vi "Search Hovered Shape.vi"(8 "error in (no error)":errorcluster, 10 "Coords":T1, 11 "Image Editor Handler in":refnum<class "Image Editor Handler.lvclass">) -> (0 "error out":errorcluster, 2 "Node ID":i32, 3 "Image Editor Handler out":refnum<class "Image Editor Handler.lvclass">)   [LabVIEW 2017, in "LV Image Editor Framework.lvlib" / "Image Editor Handler.lvclass"]
uses:
  <vilib>/LIEF/Image Editor Handler/Image Editor Handler.lvclass
  <vilib>/Utility/miscctls.llb/LVPoint32TypeDef.ctl
  <vilib>/LIEF/Image Editor Handler/Image Editor Handler.lvclass/Image Editor Handler.ctl
  <vilib>/LIEF/Forms/Shape/Shape.lvclass
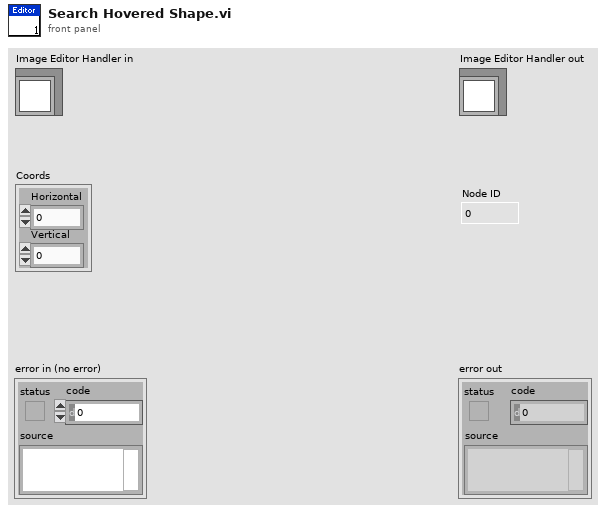
[diagram p1: front panel]
types:
  T1 = typedef "LVPoint32TypeDef.ctl" = cluster{"Horizontal":i32, "Vertical":i32}
  T2 = typedef "LVPositionTypeDef.ctl" = cluster{"Left":i32, "Top":i32}
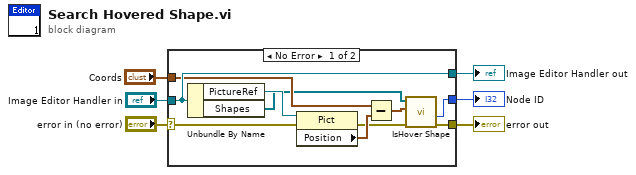
[diagram p0: block diagram]
diagram:
  n1 = case shown="No Error" "error in (no error)" {
    selector: "error in (no error)" -> [w7 w18]
    tunnel: [w10 w18] -> w5
    tunnel: [w16 w17] -> w3
    tunnel: "Image Editor Handler in" -> [w16 w17]
    tunnel: "Coords" -> [w14 _]
    tunnel: [w9 _] -> w1
    frame No Error {
      n2 = Unbundle By Name(w16) -> ("PictureRef"=w15:refnum<vi>, "Shapes"=w12:refnum<data-value>[])
      n3 = property class="Pict"(reference=w15, error in=w7) -> (error out=w8:errorcluster, "Position"=w13:T2)  [unwired: 1 out]
      n4 = Subtract(x=w14, y=w13) -> (x-y=w11:T1)
      n5 = call <vilib>:"IsHover Shape.vi"("error in (no error)"=w8, "Coords"=w11, "Shape in"=w12) -> ("error out"=w10:errorcluster, "Node ID"=w9:i32)  [unwired: 3 in, 4 out]
    }
    frame Error {
    }
  }
  "error out" <- w5
  "Image Editor Handler out" <- w3
  "Node ID" <- w1
